vi "Unwap Image.vi"() -> ()   [LabVIEW 2014]
doc: "Use this template to build a VI to use as a subVI."
uses:
  <vilib>/vision/NI_Vision_Development_Module.lvlib
panel:
  out "Src":T1(plugin-control)
  out "Dst":T1(plugin-control)
  # ":: MVi Framework V1.0 ::\nAuthor:Gaoke Yang\nEmail: gaoke.yang@yahoo.com\nWeb: www.mvicontrol.com\nCopyright (C) 2015, MVI Technologies All Rights Reserved"
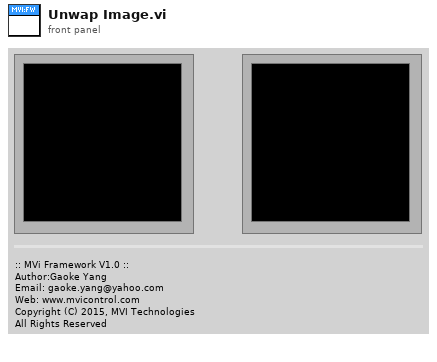
[diagram p1: front panel]
types:
  T1 = typedef "IMAQ Image.ctl" = refnum<image>
  T2 = typedef "IMAQ Circle" = cluster{"Center X":i32, "Center Y":i32, "Inner Radius":i32, "Outer Radius":i32, "Start Angle":dbl, "End Angle":dbl}
  T3 = typedef "Image Type" = u32
  T4 = typedef "ROI Descriptor" = cluster{"Global Rectangle":i32[], "Contours":cluster{"ID":enum32{"External", "Internal"}, "Type":u32, "Coordinates":i32[]}[]}
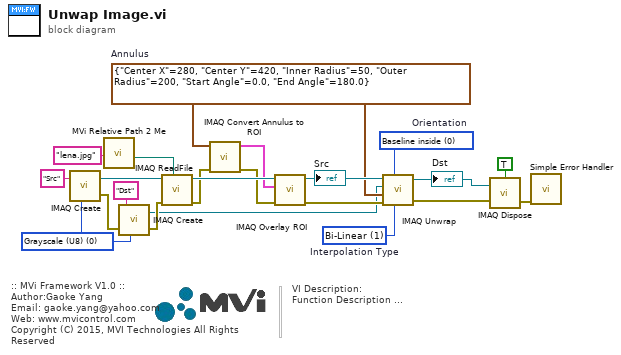
[diagram p0: block diagram]
diagram:
  w8 = u32 1 items=["Zero Order", "Bi-Linear", "Quadratic", "Cubic Spline"]  # Interpolation Type
  w12 = u32 0 items=["Baseline inside", "Baseline outside"]  # Orientation
  w5 = T2 {"Center X"=280, "Center Y"=420, "Inner Radius"=50, "Outer Radius"=200, "Start Angle"=0.0, "End Angle"=180.0}  # Annulus
  w16 = T3 0 items=["Grayscale (U8)", "Grayscale (I16)", "Grayscale (SGL)", "Complex (CSG)", "RGB (U32)", "HSL (U32)", "RGB (U64)", "Grayscale (U16)"] ("Image Type")
  # "VI Description:\nFunction Description ..."
  # ":: MVi Framework V1.0 ::\nAuthor:Gaoke Yang\nEmail: gaoke.yang@yahoo.com\nWeb: www.mvicontrol.com\nCopyright (C) 2015, MVI Technologies All Rights Reserved"
  n1 = call "IMAQ Create"("Image Name"="Src" ("name or relative path"), "Image Type"=w16) -> ("New Image"=w13:T1, "error out"=w15:errorcluster)  [unwired: 2 in, 1 out]
  n2 = call "MVi Relative Path 2 Me.vi"("Relative Path"="lena.jpg" ("name or relative path")) -> ("Appended Dir"=w18:path)  [unwired: 5 in, 1 out]
  n3 = call "IMAQ Create"("Image Name"="Dst" ("name or relative path"), "Image Type"=w16, "error in (no error)"=w15) -> ("New Image"=w1:T1, "error out"=w14:errorcluster)  [unwired: 1 in, 1 out]
  n4 = call "IMAQ ReadFile"("File Path"=w18, "error in (no error)"=w14, "Image"=w13) -> ("error out"=w7:errorcluster, "Image Out"=w11:T1)  [unwired: 4 in, 3 out]
  n5 = call "IMAQ Convert Annulus to ROI"("error in (no error)"=w7, "Annulus"=w5) -> ("error out"=w6:errorcluster, "ROI Descriptor"=w10:T4)  [unwired: 7 in]
  n6 = call "IMAQ Overlay ROI"("error in (no error)"=w6, "ROI Descriptor"=w10, "Image"=w11) -> ("error out"=w4:errorcluster, "Image Out"=w9:T1)  [unwired: 7 in]
  "Src" <- w9
  n7 = call "IMAQ Unwrap"("Image Src"=w9, "Orientation"=w12, "Image Dst"=w1, "Annulus"=w5, "Interpolation Type"=w8, "error in (no error)"=w4) -> ("Image Dst Out"=w3:T1, "error out"=w2:errorcluster)  [unwired: 1 in]
  "Dst" <- w3
  n8 = call "IMAQ Dispose"("All Images? (No)"=TRUE, "Image"=w3, "error in (no error)"=w2) -> ("error out"=w19:errorcluster)  [unwired: 3 out]
  n9 = call <vilib>:"Simple Error Handler.vi"("error in (no error)"=w19) -> ()  [unwired: 1 in, 8 out]
